vi "No Channel Wire Demo.vi"() -> ()   [LabVIEW 2022 SP3]
uses:
  Enclave/Element.ctl
  Enclave/Lossless/Lossless.lvclass/Lossless.ctl
  Enclave/Enclave/Enclave.lvclass
  Enclave/Writer/Writer.lvclass
  Enclave/Event/Event.lvclass
  Enclave/Lossless/Lossless.lvclass
  Enclave/Tag/Tag.lvclass
  Enclave/Enclave.lvlib
panel:
  out "Lossy":dbl(graph)
  out "Lossless":dbl(graph)
  out "Event":dbl(graph)
  in  "To Write":T1
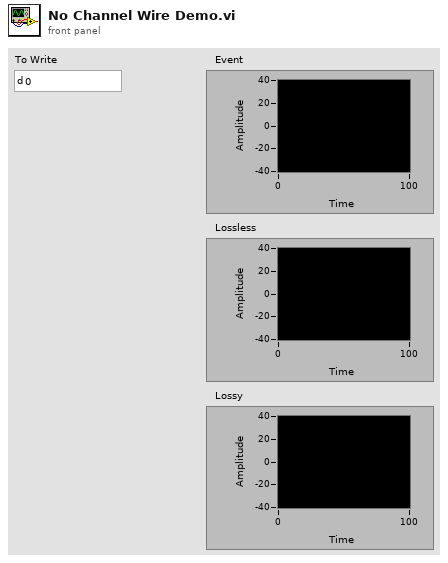
[diagram p1: front panel]
types:
  T1 = typedef "Enclave.lvlib/Element.ctl" = dbl
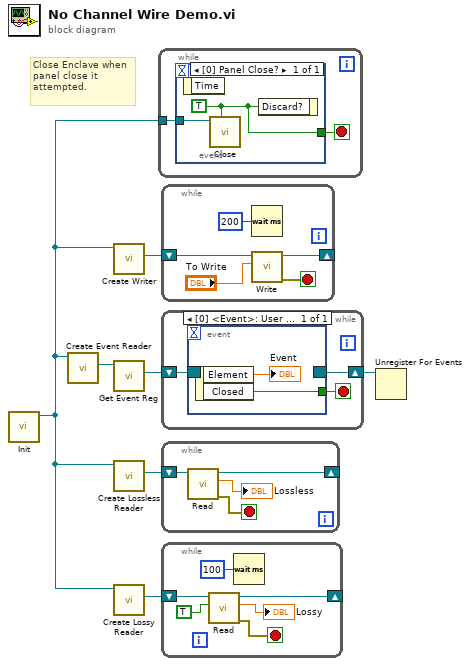
[diagram p0: block diagram]
diagram:
  # "Close Enclave when panel close it attempted."
  n1 = call "Init.vi"() -> ("Enclave out"=w1:refnum<class "Enclave.lvclass">)  [unwired: 10 in, 1 out]
  n2 = call "Create Event Reader.vi"("Enclave in"=w1) -> ("Event"=w6:refnum<class "Event.lvclass">)  [unwired: 8 in, 2 out]
  n3 = call "Create Writer.vi"("Enclave in"=w1) -> ("Writer"=w7:refnum<class "Writer.lvclass">)  [unwired: 8 in, 2 out]
  n4 = call "Get Event Reg.vi"("Event in"=w6) -> ("Event Reg"=w5:refnum<event-registration>)  [unwired: 8 in, 2 out]
  n5 = call "Create Lossless Reader.vi"("Enclave in"=w1) -> ("Lossless"=w3:refnum<class "Lossless.lvclass">)  [unwired: 8 in, 2 out]
  n6 = call "Create Lossy Reader.vi"("Enclave in"=w1) -> ("Lossy Reader"=w2:refnum<class "Tag.lvclass">)  [unwired: 8 in, 2 out]
  n7 = while {
    tunnel: w1 -> [w9]
    stop <- w8 stop-if-true
    n8 = event shown="[0] Panel Close?" {
      selector: _ -> [_]
      dyn-events: _ -> [_]
      timeout: _ -> [_]
      tunnel: w9 -> [w11]
      tunnel: [w10] -> w8
      event Panel Close? {
        w10 = TRUE ("Discard?")
        n9 = event-data() -> ()  [unwired: 1 in, 1 out]
        n10 = call "Close.vi"("Abort (F)"=w10, "Enclave in"=w11) -> ()  [unwired: 9 in, 1 out]
        n11 = event-data("Discard?"=w10) -> ()  [unwired: 1 in, 1 out]
      }
    }
  }
  n12 = while {
    shift-right: [w14] -> _
    shift-left: w7 -> [w16]
    stop <- w13 stop-if-true
    n13 = Wait (ms)(milliseconds to wait=u32 200) -> ()  [unwired: 1 out]
    n14 = call "Write.vi"("Element"="To Write", "Writer in"=w16) -> ("error out"=w13:errorcluster, "Writer out"=w14:refnum<class "Writer.lvclass">)  [unwired: 7 in, 1 out]
  }
  n15 = while {
    shift-right: [w17] -> w4
    shift-left: w5 -> [w19]
    stop <- w18 stop-if-true
    n16 = event shown="[0] <Event>: User Event" {
      selector: w19 -> [_]
      dyn-events: [_] -> w17
      timeout: _ -> [_]
      tunnel: [w21] -> w18
      event User Event {
        n17 = event-data() -> ("Element"=→"Event":T1, "Closed"=w21:bool)  [unwired: 1 in]
      }
    }
  }
  n18 = while {
    shift-right: [w22] -> _
    shift-left: w3 -> [w25]
    stop <- w24 stop-if-true
    n19 = call "Read.vi"("Lossless in"=w25) -> ("error out"=w24:errorcluster, "Element"=→"Lossless":T1, "Lossless out"=w22:refnum<class "Lossless.lvclass">)  [unwired: 7 in, 1 out]
  }
  n20 = while {
    shift-right: [w27] -> _
    shift-left: w2 -> [w31]
    stop <- w29 stop-if-true
    n21 = call "Read.vi"("ignore previous (F)"=TRUE, "Tag in"=w31) -> ("error out"=w29:errorcluster, "Element"=→"Lossy":T1, "Tag out"=w27:refnum<class "Tag.lvclass">)  [unwired: 3 in, 4 out]
    n22 = Wait (ms)(milliseconds to wait=u32 100) -> ()  [unwired: 1 out]
  }
  n23 = Unregister For Events(event registration refnum=w4) -> ()  [unwired: 1 in, 1 out]
